vi "MatrixDUTSwitch.vi"(8 "error in (no error)":errorcluster, 10 "DUT #":i32, 11 "KE3700A in":refnum<class "KE3706A.lvclass">) -> (0 "error out":errorcluster, 3 "KE3700A out":refnum<class "KE3706A.lvclass">)   [LabVIEW 2018, in "KE3706A.lvclass"]
uses:
  KE3706A.lvclass
  additional LV libraries/Keithley 3706/Keithley 3700 Series.lvlib
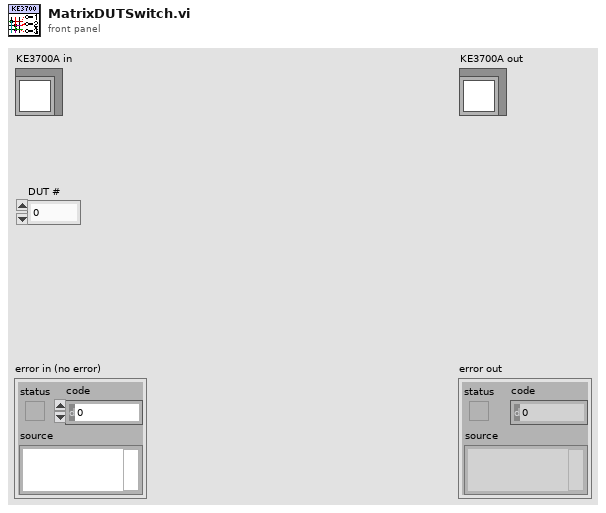
[diagram p1: front panel]
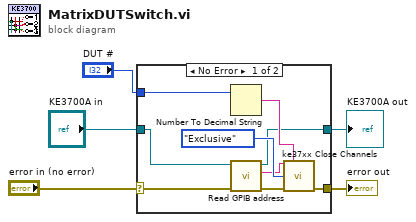
[diagram p0: block diagram]
diagram:
  n1 = case shown="No Error" "error in (no error)" {
    selector: "error in (no error)" -> [w11 w16]
    tunnel: [w7 w16] -> w4
    tunnel: "KE3700A in" -> [w12 w15]
    tunnel: [w6 w15] -> w2
    tunnel: "DUT #" -> [w14 _]
    frame No Error {
      n2 = Number To Decimal String(number=w14) -> (decimal integer string=w8:string)  [unwired: 1 in]
      n3 = call-dynamic "Read GPIB address.vi"("error in (no error)"=w11, "InstControl in"=w12) -> ("error out"=w10:errorcluster, "GPIB address"=w9:string, "InstControl out"=w6:refnum<class "KE3706A.lvclass">)  [unwired: 7 in]
      n4 = call "ke37xx Close Channels.vi"("VISA Resource Name"=w9, "Channel List"=w8, "Mode (0: Normal)"=enum16{"Normal", "Exclusive", "Slot Exclusive"}."Exclusive", "error in (no error)"=w10) -> ("error out"=w7:errorcluster)  [unwired: 10 in, 1 out]
    }
    frame Error {
    }
  }
  "error out" <- w4
  "KE3700A out" <- w2
